vi "GainScheduler.vi"(6 "LockSetpoint":bool=TRUE, 7 "On Bert?":bool=TRUE, 8 "Stacker Height":dbl format="%#_13g", 9 "Travel Direction Up":bool, 10 "StackerState":T4, 11 "Number of Totes":u8) -> (2 "Stacker Gains Out":T3)   [LabVIEW 2014]
uses:
  Typedefs/StackerStates.ctl
panel:
  in  "Bert Hover Gains":T1(array[cluster])=[{"Arm_kP"=0.35, "Arm_kI"=0.15, "Arm_kD"=0.02}, {"Arm_kP"=0.35, "Arm_kI"=0.15, "Arm_kD"=0.02}, {"Arm_kP"=0.1, "Arm_kI"=0.1, "Arm_kD"=0.02}, {"Arm_kP"=0.1, "Arm_kI"=0.1, "Arm_kD"=0.02}, {"Arm_kP"=0.1, "Arm_kI"=0.1, "Arm_kD"=0.02}, {"Arm_kP"=0.1, "Arm_kI"=0.09999999999999998, "Arm_kD"=0.02}, {"Arm_kP"=0.1, "Arm_kI"=0.1, "Arm_kD"=0.02}]
  in  "Ernie Hover Gains":T1(array[cluster])=[{"Arm_kP"=0.1, "Arm_kI"=0.1, "Arm_kD"=0.02}, {"Arm_kP"=0.1, "Arm_kI"=0.1, "Arm_kD"=0.02}, {"Arm_kP"=0.1, "Arm_kI"=0.1, "Arm_kD"=0.02}, {"Arm_kP"=0.1, "Arm_kI"=0.1, "Arm_kD"=0.02}, {"Arm_kP"=0.1, "Arm_kI"=0.1, "Arm_kD"=0.02}, {"Arm_kP"=0.1, "Arm_kI"=0.1, "Arm_kD"=0.02}, {"Arm_kP"=0.1, "Arm_kI"=0.1, "Arm_kD"=0.02}]
  in  "Ernie DropStack Gains":T1(array[cluster])=[{"Arm_kP"=0.15, "Arm_kI"=0.3, "Arm_kD"=0.015}, {"Arm_kP"=0.15, "Arm_kI"=0.3, "Arm_kD"=0.015}, {"Arm_kP"=0.15, "Arm_kI"=0.3, "Arm_kD"=0.015}, {"Arm_kP"=0.15, "Arm_kI"=0.3, "Arm_kD"=0.015}, {"Arm_kP"=0.15, "Arm_kI"=0.3, "Arm_kD"=0.015}, {"Arm_kP"=0.15, "Arm_kI"=0.3, "Arm_kD"=0.015}, {"Arm_kP"=0.15, "Arm_kI"=0.3, "Arm_kD"=0.015}]
  in  "Bert DropStack Gains":T1(array[cluster])=[{"Arm_kP"=0.12, "Arm_kI"=0.3, "Arm_kD"=0.015}, {"Arm_kP"=0.12, "Arm_kI"=0.3, "Arm_kD"=0.015}, {"Arm_kP"=0.12, "Arm_kI"=0.3, "Arm_kD"=0.015}, {"Arm_kP"=0.12, "Arm_kI"=0.3, "Arm_kD"=0.018}, {"Arm_kP"=0.12, "Arm_kI"=0.3, "Arm_kD"=0.015}, {"Arm_kP"=0.12, "Arm_kI"=0.3, "Arm_kD"=0.015}, {"Arm_kP"=0.15, "Arm_kI"=0.3, "Arm_kD"=0.015}]
  in  "Lock Gains":T2={"Arm_kP"=0.5, "Arm_kI"=0.0, "Arm_kD"=0.0}
  in  "Ernie Blow Through Bottom Gains":T1(array[cluster])=[{"Arm_kP"=1.2, "Arm_kI"=0.0, "Arm_kD"=0.0}, {"Arm_kP"=1.2, "Arm_kI"=0.0, "Arm_kD"=0.0}, {"Arm_kP"=2.3, "Arm_kI"=0.0, "Arm_kD"=0.0}, {"Arm_kP"=2.5, "Arm_kI"=0.0, "Arm_kD"=0.0}, {"Arm_kP"=2.6, "Arm_kI"=0.0, "Arm_kD"=0.0}, {"Arm_kP"=2.5, "Arm_kI"=0.0, "Arm_kD"=0.0}, {"Arm_kP"=0.5, "Arm_kI"=0.0, "Arm_kD"=0.0}]
  in  "Bert Blow Through Bottom Gains":T1(array[cluster])=[{"Arm_kP"=1.2, "Arm_kI"=0.1, "Arm_kD"=0.0}, {"Arm_kP"=1.2, "Arm_kI"=0.1, "Arm_kD"=0.02}, {"Arm_kP"=1.45, "Arm_kI"=0.1, "Arm_kD"=0.02}, {"Arm_kP"=1.45, "Arm_kI"=0.1, "Arm_kD"=0.01}, {"Arm_kP"=1.45, "Arm_kI"=0.2, "Arm_kD"=0.01}, {"Arm_kP"=1.45, "Arm_kI"=0.2, "Arm_kD"=0.01}, {"Arm_kP"=0.5, "Arm_kI"=0.2, "Arm_kD"=0.0}]
  in  "Ernie Stacker Gain Scheduler Up":T1(array[cluster])=[{"Arm_kP"=0.1, "Arm_kI"=0.1, "Arm_kD"=0.018}, {"Arm_kP"=0.1, "Arm_kI"=0.1, "Arm_kD"=0.018}, {"Arm_kP"=0.18, "Arm_kI"=0.15, "Arm_kD"=0.02}, {"Arm_kP"=0.11, "Arm_kI"=0.2, "Arm_kD"=0.02}, {"Arm_kP"=0.15, "Arm_kI"=0.6, "Arm_kD"=0.02}, {"Arm_kP"=0.15, "Arm_kI"=0.6, "Arm_kD"=0.02}, {"Arm_kP"=0.3, "Arm_kI"=0.7, "Arm_kD"=0.01}]
  in  "Ernie Stacker Gain Scheduler Down":T1(array[cluster])=[{"Arm_kP"=0.2, "Arm_kI"=0.4, "Arm_kD"=0.015}, {"Arm_kP"=0.2, "Arm_kI"=0.4, "Arm_kD"=0.015}, {"Arm_kP"=0.5, "Arm_kI"=1.5, "Arm_kD"=0.02}, {"Arm_kP"=0.5, "Arm_kI"=0.8, "Arm_kD"=0.02}, {"Arm_kP"=0.15, "Arm_kI"=0.8, "Arm_kD"=0.02}, {"Arm_kP"=0.15, "Arm_kI"=0.8, "Arm_kD"=0.02}, {"Arm_kP"=0.1, "Arm_kI"=0.8, "Arm_kD"=0.02}]
  in  "Bert Stacker Gain Scheduler Up":T1(array[cluster])=[{"Arm_kP"=0.2, "Arm_kI"=0.0, "Arm_kD"=0.012}, {"Arm_kP"=0.2, "Arm_kI"=0.0, "Arm_kD"=0.012}, {"Arm_kP"=0.2, "Arm_kI"=0.5, "Arm_kD"=0.012}, {"Arm_kP"=0.2, "Arm_kI"=0.5, "Arm_kD"=0.012}, {"Arm_kP"=0.2, "Arm_kI"=0.6, "Arm_kD"=0.012}, {"Arm_kP"=0.2, "Arm_kI"=0.65, "Arm_kD"=0.012}, {"Arm_kP"=0.3, "Arm_kI"=0.8, "Arm_kD"=0.01}]
  in  "Bert Stacker Gain Scheduler Down":T1(array[cluster])=[{"Arm_kP"=0.3, "Arm_kI"=0.0, "Arm_kD"=0.015}, {"Arm_kP"=0.3, "Arm_kI"=0.0, "Arm_kD"=0.015}, {"Arm_kP"=0.3, "Arm_kI"=0.0, "Arm_kD"=0.015}, {"Arm_kP"=0.25, "Arm_kI"=0.0, "Arm_kD"=0.02}, {"Arm_kP"=0.25, "Arm_kI"=0.0, "Arm_kD"=0.02}, {"Arm_kP"=0.25, "Arm_kI"=0.0, "Arm_kD"=0.02}, {"Arm_kP"=0.25, "Arm_kI"=0.0, "Arm_kD"=0.0}]
  # "Since these are two separate mechanisms, they should move into two separate VIs\nAnd the VI should go within the mechanism code"
  # "0 was:\n.3\n1"
  # "1 was:\n.15\n.8"
  # "Again make more generic"
  # "currently disabled"
  # "Number of Totes:        0                     1                       2                       3                      4                       5                       6"
  # "Number of Totes:        0                     1                       2                       3                      4                       5                       6"
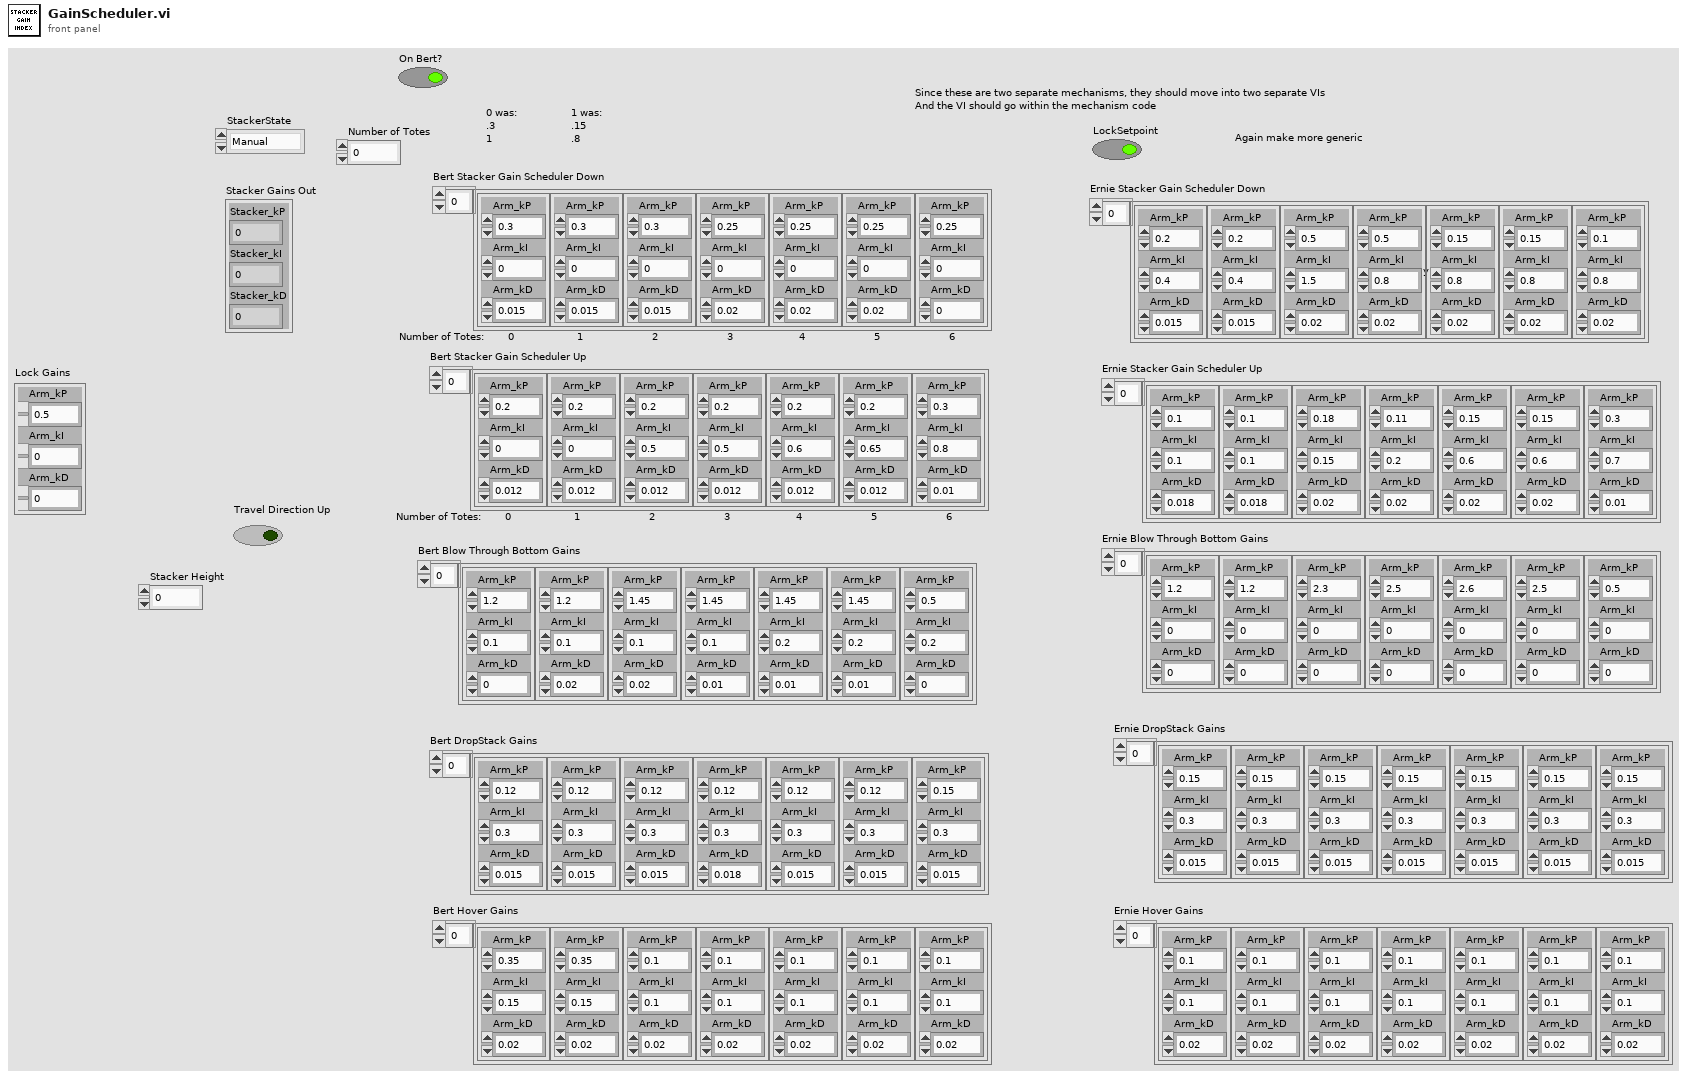
[diagram p1: front panel]
types:
  T1 = cluster{"Arm_kP":dbl, "Arm_kI":dbl, "Arm_kD":dbl}[]
  T2 = cluster{"Arm_kP":dbl, "Arm_kI":dbl, "Arm_kD":dbl}
  T3 = cluster{"Stacker_kP":dbl, "Stacker_kI":dbl, "Stacker_kD":dbl}
  T4 = typedef "StackerStates.ctl" = enum16{"Manual ", "Hold", "Hold5", "Hold6", "GetTote", "DropStack", "Hover", "Hover5", "Wait for Up", "DecideHold", "DownTimerPeriod", "Prep Intake for Drop", "Check Arm before 5", "Make Arm ready for 5", "Check Arm before 6", "Make Arm ready for 6", "Delay for 5", "Delay for 6"}
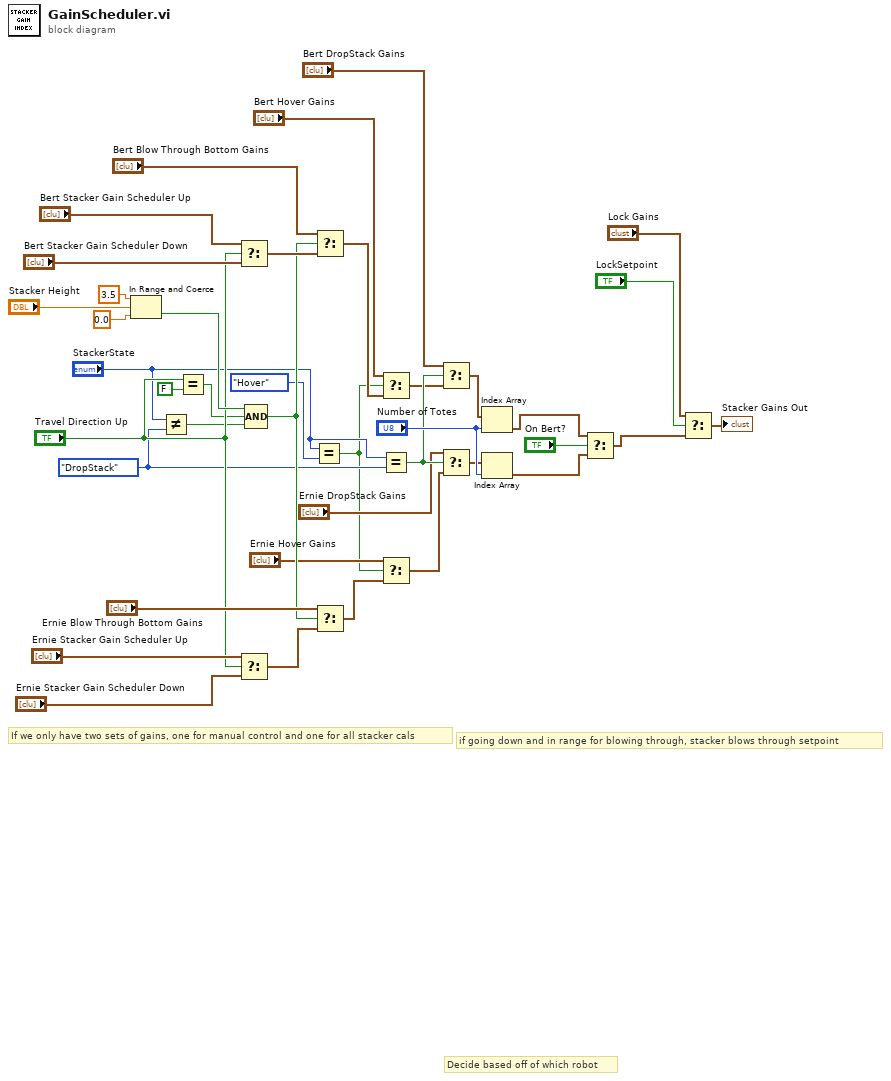
[diagram p0: block diagram]
diagram:
  w16 = StackerStates."DropStack" ("y")
  # "if going down and in range for blowing through, stacker blows through setpoint"
  # "Decide based off of which robot"
  # "If we only have two sets of gains, one for manual control and one for all stacker cals"
  n1 = In Range and Coerce(upper limit=3.5, x="Stacker Height", lower limit=0.0) -> (In Range?=w26:bool)  [unwired: 1 out]
  n2 = Not Equal?(x="StackerState", y=w16) -> (x != y?=w17:bool)
  n3 = Equal?(x="Travel Direction Up", y=FALSE) -> (x = y?=w22:bool)
  n4 = Select(t="Bert Stacker Gain Scheduler Up", s="Travel Direction Up", f="Bert Stacker Gain Scheduler Down") -> (s? t:f=w29:T1)
  n5 = Select(t="Ernie Stacker Gain Scheduler Up", s="Travel Direction Up", f="Ernie Stacker Gain Scheduler Down") -> (s? t:f=w27:T1)
  n6 = Compound Arithmetic op=AND(w26, w22, w17) -> (w21:bool)
  n7 = Equal?(x="StackerState", y=StackerStates."Hover") -> (x = y?=w2:bool)
  n8 = Select(t="Bert Blow Through Bottom Gains", s=w21, f=w29) -> (s? t:f=w4:T1)
  n9 = Select(t="Ernie Blow Through Bottom Gains", s=w21, f=w27) -> (s? t:f=w7:T1)
  n10 = Select(t="Bert Hover Gains", s=w2, f=w4) -> (s? t:f=w3:T1)
  n11 = Equal?(x="StackerState", y=w16) -> (x = y?=w13:bool)
  n12 = Select(t="Ernie Hover Gains", s=w2, f=w7) -> (s? t:f=w6:T1)
  n13 = Select(t="Bert DropStack Gains", s=w13, f=w3) -> (s? t:f=w14:T1)
  n14 = Select(t="Ernie DropStack Gains", s=w13, f=w6) -> (s? t:f=w11:T1)
  n15 = Index Array(array=w14, index="Number of Totes") -> (element=w38:T2)
  n16 = Index Array(array=w11, index="Number of Totes") -> (element=w36:T2)
  n17 = Select(t=w38, s="On Bert?", f=w36) -> (s? t:f=w1:T2)
  n18 = Select(t="Lock Gains", s="LockSetpoint", f=w1) -> (s? t:f=→"Stacker Gains Out":T2)
